vi "Initialize Thread.vi"(8 "error in (no error)":errorcluster, 10 "thread settings":T1, 11 "UDP Transceiver in":refnum<class "UDP Transceiver.lvclass">) -> (0 "error out":errorcluster, 3 "UDP Transceiver out":refnum<class "UDP Transceiver.lvclass">)   [LabVIEW 2017, in "UDP.lvlib" / "UDP Transceiver.lvclass"]
uses:
  UDP Transceiver.lvclass
  Builds/Data Sharing Framework/Current/Core/DSF Core.lvlibp/Typedefs/DSF Settings Info.ctl
  UDP Transceiver.lvclass/UDP Transceiver.ctl
  UDP Invalid Setting.vi
  Builds/Data Sharing Framework/Current/Core/DSF Core.lvlibp/Classes/Configuration/Configuration Session.lvclass
  Builds/Data Sharing Framework/Current/Core/DSF Core.lvlibp
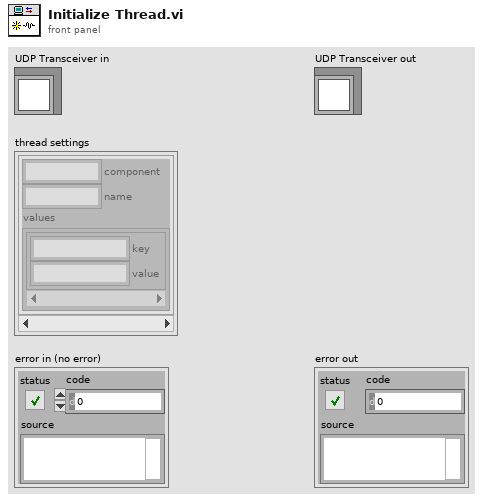
[diagram p1: front panel]
types:
  T1 = typedef "DSF Core.lvlibp/DSF Settings Info.ctl" = cluster{"component":string, "name":string, "values":cluster{"key":string, "value":string}[]}[]
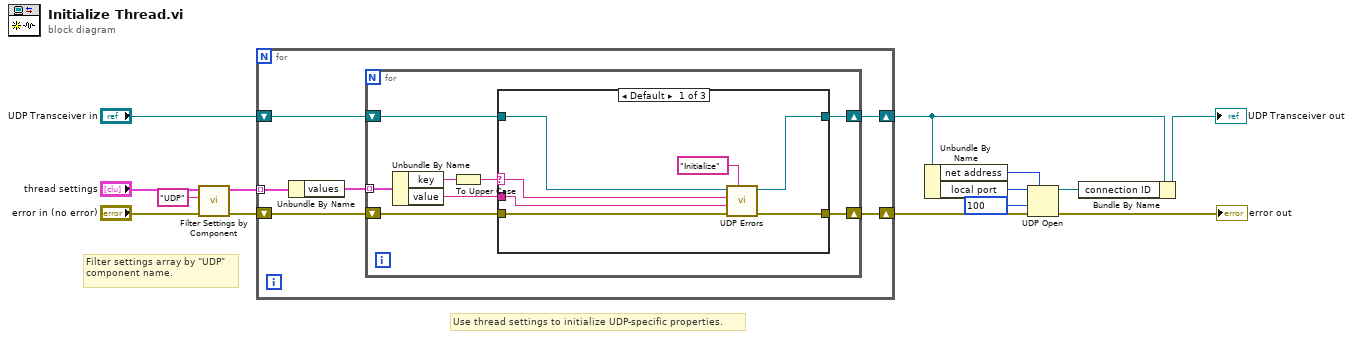
[diagram p0: block diagram]
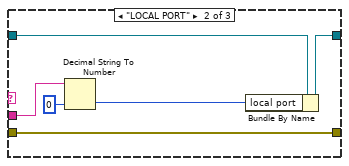
[diagram p2: hidden frame]
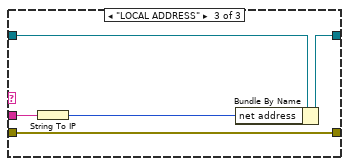
[diagram p3: hidden frame]
diagram:
  # "Filter settings array by \"UDP\" component name."
  # "Use thread settings to initialize UDP-specific properties."
  n1 = call "Filter Settings by Component.vi"("error in (no error)"="error in (no error)", "component"="UDP", "settings"="thread settings") -> ("error out"=w12:errorcluster, "filtered settings"=w14:T1)  [unwired: 7 in]
  n2 = for {
    tunnel: w14 -> [w16] mode=indexing
    shift-right: [w19] -> w2
    shift-left: "UDP Transceiver in" -> [w20]
    shift-right: [w17] -> w4
    shift-left: w12 -> [w18]
    n3 = Unbundle By Name(w16) -> ("values"=w15:cluster{"key":string, "value":string}[])
    n4 = for {
      shift-right: [w27] -> w19
      shift-left: w20 -> [w28]
      shift-right: [w25] -> w17
      shift-left: w18 -> [w26]
      tunnel: w15 -> [w24] mode=indexing
      n5 = Unbundle By Name(w24) -> ("key"=w22:string, "value"=w23:string)
      n6 = To Upper Case(1:w22) -> (0:w21:string)
      n7 = case shown="Default" w21 {
        selector: w21 -> [w33 _ _]
        tunnel: w28 -> [w32 w36 w46]
        tunnel: [w31 w40 w45] -> w27
        tunnel: w26 -> [w35 w39 w44]
        tunnel: [w34 w39 w44] -> w25
        tunnel: w23 -> [w29 w37 w42]
        frame Default {
          n8 = call-poly "UDP Errors.vi"("source vi name"="Initialize", "error in (no error)"=w35, "value"=w29, "key"=w33, "UDP in"=w32) -> ("error out"=w34:errorcluster, "UDP out"=w31:refnum<class "UDP Transceiver.lvclass">)  [unwired: 5 in]
        }
        frame "LOCAL PORT" {
          n9 = Decimal String To Number(string=w37, default (0L)=u16 0 ("default (0 I32)")) -> (number=w38:u16)  [unwired: 1 in, 1 out]
          n10 = Bundle By Name(cluster=w36, "local port"=w38) -> (w40:refnum<class "UDP Transceiver.lvclass">)
        }
        frame "LOCAL ADDRESS" {
          n11 = String To IP(1:w42) -> (0:w43:u32)
          n12 = Bundle By Name(cluster=w46, "net address"=w43) -> (w45:refnum<class "UDP Transceiver.lvclass">)
        }
      }
    }
  }
  n13 = Unbundle By Name(w2) -> ("net address"=w5:u32, "local port"=w8:u16)
  n14 = UDP Open(7:w5, 8:w4, 9:100 ("timeout ms (25000)"), 11:w8) -> (port=w6:refnum<k16>, 0:→"error out":errorcluster)  [unwired: 1 in, 1 out]
  n15 = Bundle By Name(cluster=w2, "connection ID"=w6) -> (→"UDP Transceiver out":refnum<class "UDP Transceiver.lvclass">)
